vi "HTML_Get_Core_RequiredDependencies.vi"() -> (1 "HTML_JS_General_Required_Dependencies":path[](array[path]), 2 "HTML_CSS_General_Required_Dependencies":path[](array[path]))   [LabVIEW 2014]
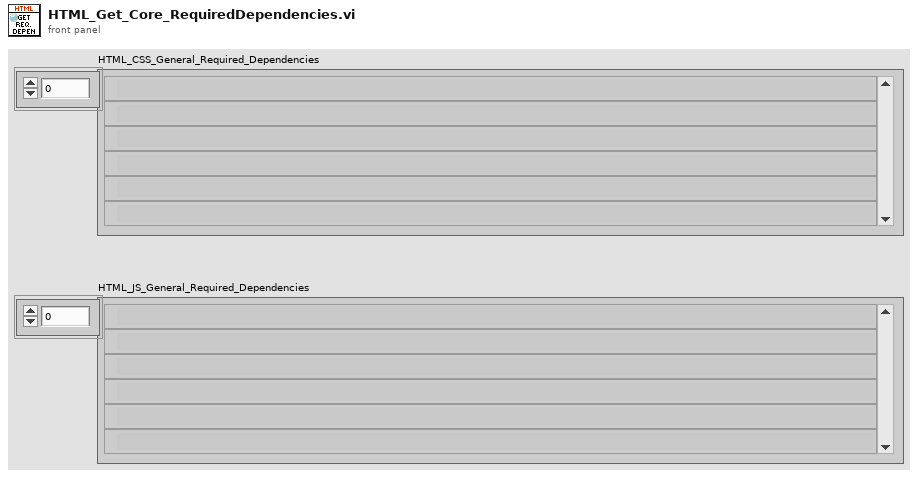
[diagram p1: front panel]
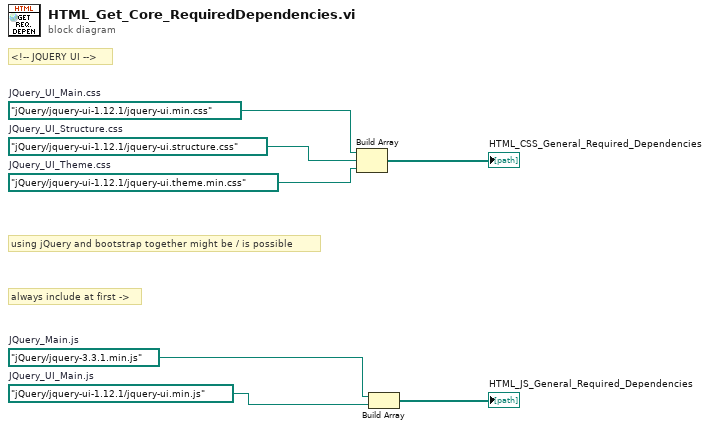
[diagram p0: block diagram]
diagram:
  w3 = path "jQuery/jquery-ui-1.12.1/jquery-ui.theme.min.css"  # JQuery_UI_Theme.css
  w5 = path "jQuery/jquery-ui-1.12.1/jquery-ui.structure.css"  # JQuery_UI_Structure.css
  w4 = path "jQuery/jquery-ui-1.12.1/jquery-ui.min.css"  # JQuery_UI_Main.css
  w7 = path "jQuery/jquery-ui-1.12.1/jquery-ui.min.js"  # JQuery_UI_Main.js
  w6 = path "jQuery/jquery-3.3.1.min.js"  # JQuery_Main.js
  # "using jQuery and bootstrap together might be / is possible"
  # "<!-- JQUERY UI -->"
  # "always include at first ->"
  n1 = Build Array(w4, w5, w3) -> (→"HTML_CSS_General_Required_Dependencies":path[])
  n2 = Build Array(w6, w7) -> (→"HTML_JS_General_Required_Dependencies":path[])
